vi "set_lag.vi"(8 "error in (no error)":errorcluster, 10 "lag":dbl[unit], 11 "DAQmxWriteSignals.lvclass in":refnum<class "SignalWriterMM140725DAQmx.lvclass">) -> (0 "error out":errorcluster, 3 "DAQmxWriteSignals.lvclass out":refnum<class "SignalWriterMM140725DAQmx.lvclass">)   [LabVIEW 2010, in "SignalWriterMM140725DAQmx.lvclass"]
uses:
  SignalWriterMM140725DAQmx.lvclass
  GenericSignalWriter/GenericSignalWriter/GenericSignalWriter.lvclass
  SignalWriterMM140725DAQmx.lvclass/SignalWriterMM140725DAQmx.ctl
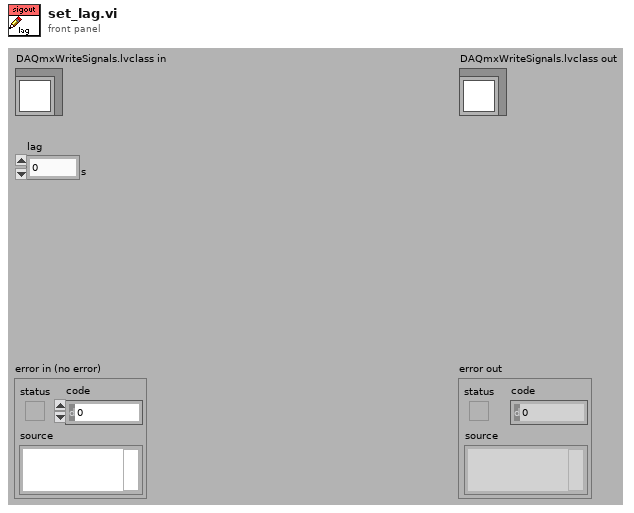
[diagram p1: front panel]
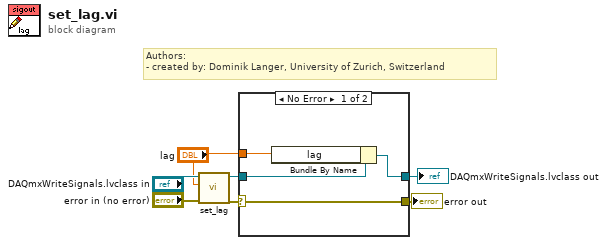
[diagram p0: block diagram]
diagram:
  # "Authors: \n- created by: Dominik Langer, University of Zurich, Switzerland"
  n1 = call-parent "set_lag.vi"("error in (no error)"="error in (no error)", "lag"="lag", "GenericWriteSignals.lvclass in"="DAQmxWriteSignals.lvclass in") -> ("error out"=w4:errorcluster, "GenericWriteSignals.lvclass out"=w2:refnum<class "SignalWriterMM140725DAQmx.lvclass">)  [unwired: 7 out]
  n2 = case shown="No Error" w4 {
    selector: w4 -> [w10 w13]
    tunnel: "lag" -> [w11 _]
    tunnel: [w10 w13] -> w3
    tunnel: [w9 w12] -> w1
    tunnel: w2 -> [w8 w12]
    frame No Error {
      n3 = Bundle By Name(cluster=w8, "lag"=w11) -> (w9:refnum<class "SignalWriterMM140725DAQmx.lvclass">)
    }
    frame Error {
    }
  }
  "error out" <- w3
  "DAQmxWriteSignals.lvclass out" <- w1
